vi "solar Msg Voyager (Packet).vi"(6 "Suppress Errors? (T)":bool=TRUE, 7 "CMD":enum8{"CMD", "TLM"}(ring), 8 "error in (no error)":errorcluster, 10 "DATA (Included HDR)":string, 11 "solar in":refnum<class "solar.lvclass">) -> (0 "error out":errorcluster, 3 "solar out":refnum<class "solar.lvclass">)   [LabVIEW 2018]
doc: "This sends the raw packet data to the Voyager interface. Use this function for customly formatted Voyager packets. The DATA must contain the header definition."
uses:
  solar.lvclass
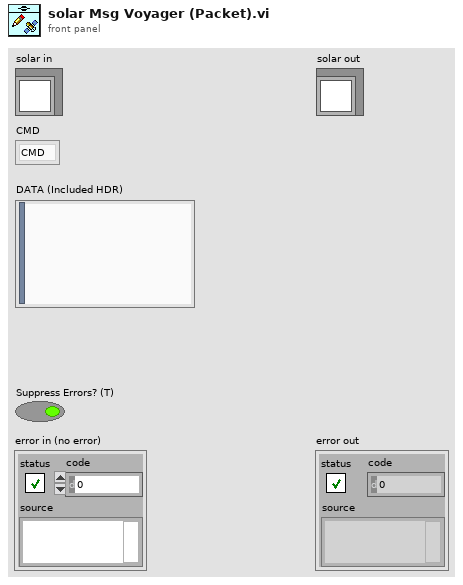
[diagram p1: front panel]
types:
  T1 = typedef "solar_voy_ctl Voyager Refnum.ctl" = refnum<k1>
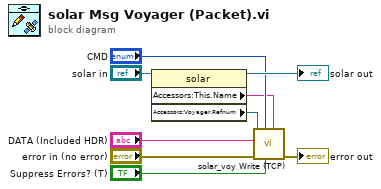
[diagram p0: block diagram]
diagram:
  n1 = property class="solar"(reference="solar in") -> (reference out=→"solar out":refnum<class "solar.lvclass">, "Accessors:This.Name"=w1:string, "Accessors:Voyager.Refnum"=w7:T1)  [unwired: 1 in, 1 out]
  n2 = call "solar_voy Write (TCP).vi"("TARGET"=w1, "Suppress Errors? (T)"="Suppress Errors? (T)", "CMD"="CMD", "error in (no error)"="error in (no error)", "TCP Data to Send"="DATA (Included HDR)", "Voyager Refnum in"=w7) -> ("error out"=→"error out":errorcluster)  [unwired: 3 in, 2 out]
